vi "AuMT8852B EDR Differential Phase Encoding Results LEG.vi"(8 "error in (no error)":errorcluster, 11 "VISA session":refnum<visa-resource-name>) -> (0 "error out":errorcluster, 2 "error code":i32, 3 "VISA session out":refnum<visa-resource-name>, 4 "Results":T1)   [LabVIEW 2017]
doc: "Anritsu MT8852B Bluetooth Tester\n\n<B>NOTE:</B> USE THIS VI ONLY FOR MT8852B FIRMWARE VERSIONS UP TO AND INCLUDING 4.08.100\n\nReturns the summary results of the EDR Differential Phase Encoding test.\n\nOUTPUT\nResults - measurements made during the test."
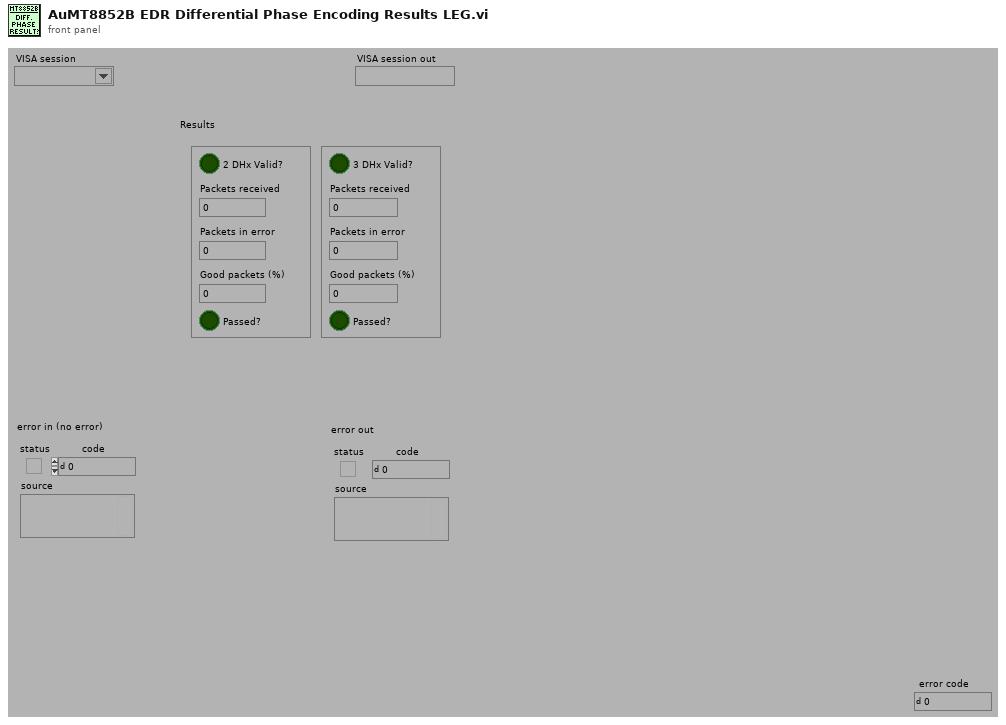
[diagram p1: front panel]
types:
  T1 = cluster{"2 DHx Valid?":bool, "Packets received":u32, "Packets in error":u32, "Passed?":bool, "Good packets (%)":u32, "3 DHx Valid?":bool, "Packets received":u32, "Packets in error":u32, "Passed?":bool, "Good packets (%)":u32}
  T2 = enum16{"Simulate", "Range check", "Cache", "Query instrument status"}
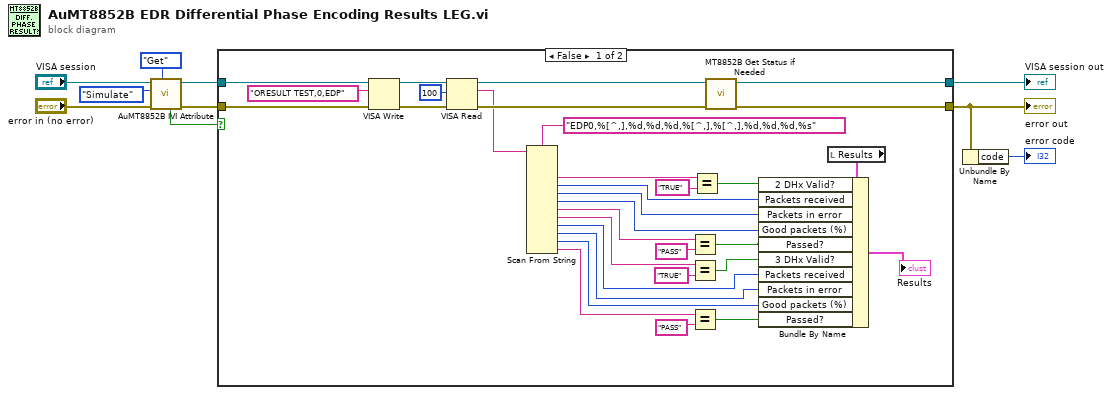
[diagram p0: block diagram]
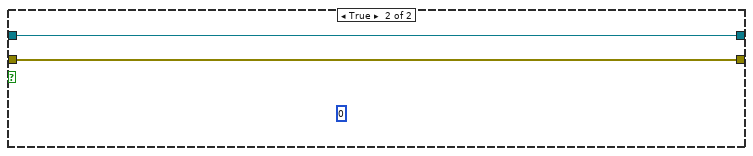
[diagram p2: hidden frame]
diagram:
  n1 = call <instrlib>:"AuMT8852B IVI Attribute.vi"("Set/Get (Set)"=enum16{"Set", "Get"}."Get", "error in (no error)"="error in (no error)", "Flag (Simulate)"=T2."Simulate", "VISA session"="VISA session") -> ("error out"=w7:errorcluster, "VISA session out"=w9:refnum<visa-resource-name>, "Value out"=w3:bool)  [unwired: 5 in]
  n2 = case shown="False" w3 {
    tunnel: [w34 w44] -> w10
    tunnel: [w33 w43] -> w1
    tunnel: w9 -> [w41 w44]
    tunnel: w7 -> [w40 w43]
    frame False {
      n3 = VISA Write(VISA resource name=w41, write buffer="ORESULT TEST,0,EDP" ("write buffer (\"\")"), error in (no error)=w40) -> (VISA resource name out=w39:refnum<visa-resource-name>, error out=w38:errorcluster)  [unwired: 1 out]
      n4 = VISA Read(VISA resource name=w39, byte count=u32 100 ("byte count (0)"), error in (no error)=w38) -> (VISA resource name out=w32:refnum<visa-resource-name>, read buffer=w30:string, error out=w31:errorcluster)  [unwired: 1 out]
      n5 = Scan From String(format string="EDP0,%[^,],%d,%d,%d,%[^,],%[^,],%d,%d,%d,%s" ("Format String"), input string=w30) -> (output 1=w29:string, output 2=w25:i32, output 3=w24:i32, output 4=w23:i32, output 5=w20:string, output 6=w17:string, output 7=w16:i32, output 8=w15:i32, output 9=w14:i32, output 10=w13:string)  [unwired: 12 in, 3 out]
      n6 = Equal?(x=w20, y="PASS") -> (x = y?=w19:bool)
      n7 = Equal?(x=w17, y="TRUE") -> (x = y?=w18:bool)
      n8 = Equal?(x=w13, y="PASS") -> (x = y?=w12:bool)
      n9 = Equal?(x=w29, y="TRUE") -> (x = y?=w26:bool)
      n10 = call <instrlib>:"MT8852B Get Status if Needed.vi"("error in (no error)"=w31, "VISA session"=w32) -> ("error out"=w33:errorcluster, "VISA session out"=w34:refnum<visa-resource-name>)  [unwired: 8 in]
      n11 = local read "Results"() -> (w27:T1)
      n12 = Bundle By Name(cluster=w27, "2 DHx Valid?"=w26, "Packets received"=w25, "Packets in error"=w24, "Good packets (%)"=w23, "Passed?"=w19, "3 DHx Valid?"=w18, "Packets received"=w16, "Packets in error"=w15, "Good packets (%)"=w14, "Passed?"=w12) -> (→"Results":T1)
    }
    frame True {
      (unwired) u8 0
    }
  }
  "error out" <- w1
  "VISA session out" <- w10
  n13 = Unbundle By Name(w1) -> ("code"=→"error code":i32)
